vi "Write Custom VI Path.vi"(8 "error in (no error)":errorcluster, 10 "Custom VI Path":path, 11 "Template in":refnum<class "MetaDataObj.lvclass">) -> (0 "error out":errorcluster, 3 "Template out":refnum<class "MetaDataObj.lvclass">)   [LabVIEW 2016, in "MetaDataObj.lvclass"]
uses:
  <resource>/dialog/NewProjectWizard/MetaDataObj/MetaDataObj.lvclass
  <resource>/dialog/NewProjectWizard/MetaDataObj/MetaDataObj.lvclass/MetaDataObj.ctl
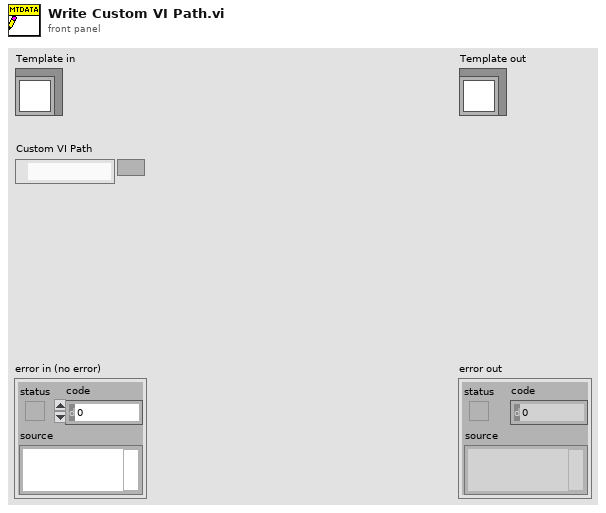
[diagram p1: front panel]
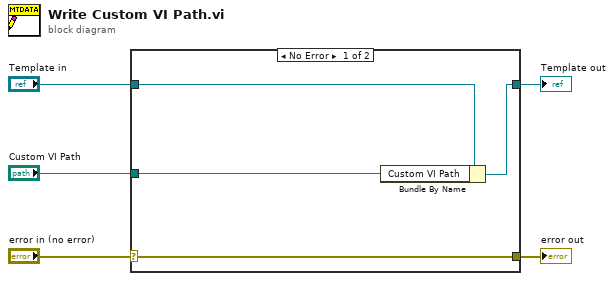
[diagram p0: block diagram]
diagram:
  n1 = case shown="No Error" "error in (no error)" {
    selector: "error in (no error)" -> [w9 w10]
    tunnel: [w9 w10] -> w4
    tunnel: [w7 w11] -> w2
    tunnel: "Template in" -> [w8 w11]
    tunnel: "Custom VI Path" -> [w6 _]
    frame No Error {
      n2 = Bundle By Name(cluster=w8, "Custom VI Path"=w6) -> (w7:refnum<class "MetaDataObj.lvclass">)
    }
    frame Error {
    }
  }
  "error out" <- w4
  "Template out" <- w2
